vi "Post Webmessage.vi"(8 "error in (no error)":errorcluster, 9 "Send as JSON":bool, 10 "Message":string, 11 "WebView2 Control in":refnum<class "WebView2 QControl.lvclass">) -> (0 "error out":errorcluster, 3 "WebView2 Control out":refnum<class "WebView2 QControl.lvclass">)   [LabVIEW 2020, in "WebView2 QControl.lvlib" / "WebView2 QControl.lvclass"]
uses:
  WebView2 QControl.lvclass
  WebView2 QControl.lvclass/WebView2 QControl.ctl
  Webview2 Lib/WebView2 Control Object/WebView2 Control.lvclass
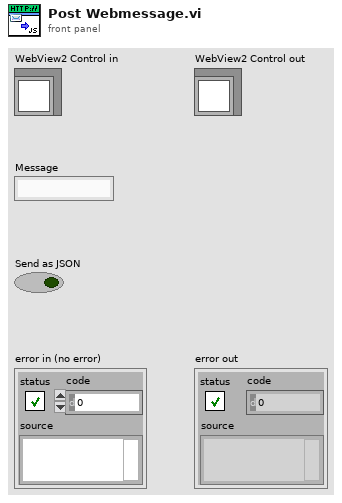
[diagram p1: front panel]
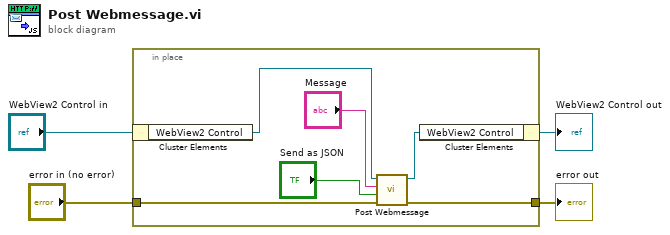
[diagram p0: block diagram]
diagram:
  n1 = in-place {
    in-place-border: "error in (no error)" -> [w10]
    in-place-border: [w9] -> w1
    n2 = in-place-cluster #1("WebView2 Control in") -> ("WebView2 Control"=w8:refnum<class "WebView2 Control.lvclass">)
    n3 = call "Post Webmessage.vi"("error in (no error)"=w10, "Send as JSON"="Send as JSON", "Message"="Message", "WebView2 Control in"=w8) -> ("error out"=w9:errorcluster, "WebView2 Control out"=w7:refnum<class "WebView2 Control.lvclass">)  [unwired: 6 in]
    n4 = in-place-cluster #1("WebView2 Control"=w7) -> (→"WebView2 Control out":refnum<class "WebView2 QControl.lvclass">)
  }
  "error out" <- w1
